vi "subfft_원본.vi"(2 "y-signal":dbl[](array[numeric]) format="%.2f", 3 "time step":dbl format="%.2f") -> (0 "Phase":cluster{"f0":dbl, "df":dbl, "real part":dbl[]} {"real part" format="%.2f"; "df" format="%.2f"; "f0" format="%.2f"}, 1 "Amplitude":cluster{"f0":dbl, "df":dbl, "real part":dbl[]} {"real part" format="%.2f"; "df" format="%.2f"; "f0" format="%.2f"})   [LabVIEW 2010]
uses:
  <vilib>/measure/maspectr.llb/FFT Spectrum (Mag-Phase) for 1 Chan.vi
  <vilib>/measure/NI_MAPro.lvlib
panel:
  in  "view":T1 caption="보기"
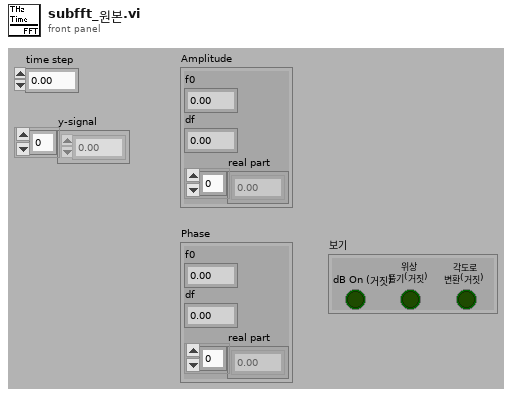
[diagram p1: front panel]
types:
  T1 = cluster{"dB On (F)":bool, "unwrap phase (F)":bool, "convert to degree (F)":bool}
  T2 = enum16{"None ", "Hanning", "Hamming", "Blackman-Harris", "Exact Blackman", "Blackman", "Flat Top", "4 Term B-Harris ", "7 Term B-Harris", "Low Sidelobe"}
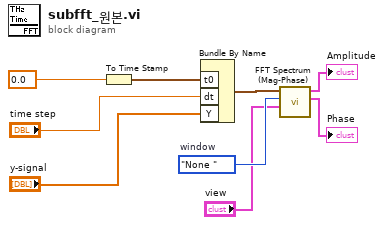
[diagram p0: block diagram]
diagram:
  w3 = T2."None "  # window
  n1 = To Time Stamp(1:0.0 ("t0")) -> (0:w2:timestamp)
  n2 = Bundle By Name("t0"=w2, "dt"="time step", "Y"="y-signal") -> (w6:waveform(dbl))  [unwired: 1 in]
  n3 = call-poly <vilib>:"FFT Spectrum (Mag-Phase).vi"("view"="view", "window"=w3, "time signal"=w6) -> ("phase"=→"Phase":cluster{"f0":dbl, "df":dbl, "phase":dbl[]}, "magnitude"=→"Amplitude":cluster{"f0":dbl, "df":dbl, "magnitude":dbl[]})  [unwired: 4 in, 3 out]
